vi "Frecuencia.vi"(8 "error in (no error)":errorcluster, 10 "Frecuencia":dbl, 11 "Generador funciones ACQ in":refnum<class "Generador funciones ACQ.lvclass">) -> (0 "error out":errorcluster, 3 "Generador funciones ACQ out":refnum<class "Generador funciones ACQ.lvclass">)   [LabVIEW 2019, in "Generador funciones ACQ.lvlib" / "Generador funciones ACQ.lvclass"]
uses:
  Generador funciones ACQ.lvclass
  Generador funciones ACQ.lvclass/Generador funciones ACQ.ctl
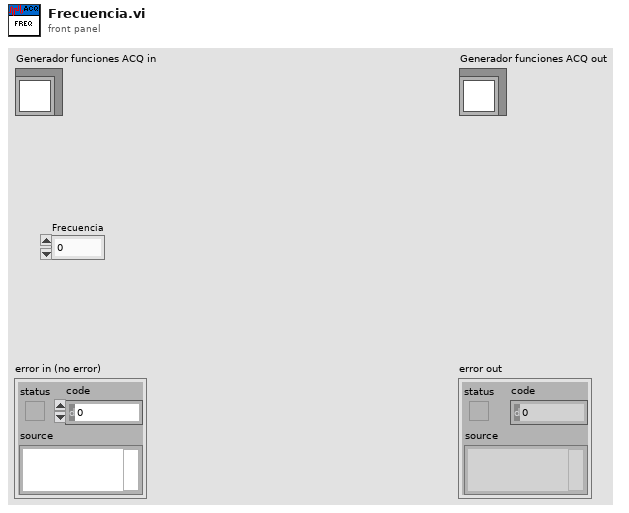
[diagram p1: front panel]
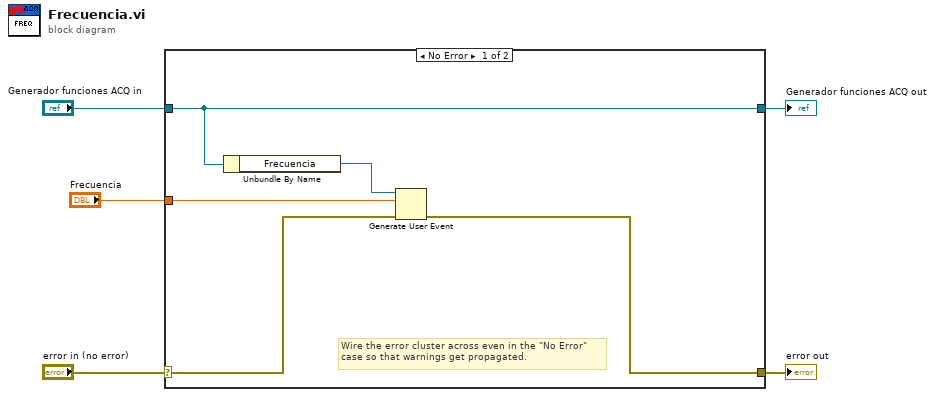
[diagram p0: block diagram]
diagram:
  n1 = case shown="No Error" "error in (no error)" {
    selector: "error in (no error)" -> [w7 w12]
    tunnel: [w6 w12] -> w4
    tunnel: [w9 w11] -> w2
    tunnel: "Generador funciones ACQ in" -> [w9 w11]
    tunnel: "Frecuencia" -> [w10 _]
    frame No Error {
      # "Wire the error cluster across even in the \"No Error\"\ncase so that warnings get propagated."
      n2 = Unbundle By Name(w9) -> ("Frecuencia"=w8:refnum<user-event>)
      n3 = Generate User Event(user event=w8, event data cluster=w10, error in=w7) -> (error out=w6:errorcluster)  [unwired: 1 in, 1 out]
    }
    frame Error {
    }
  }
  "error out" <- w4
  "Generador funciones ACQ out" <- w2
